vi "Sort_String_Array.vi"(0 "Unsorted String":string[](array[string])) -> (1 "Sorted String":string[](array[string]), 2 "Array 2":dbl[](array[numeric]))   [LabVIEW 2014]
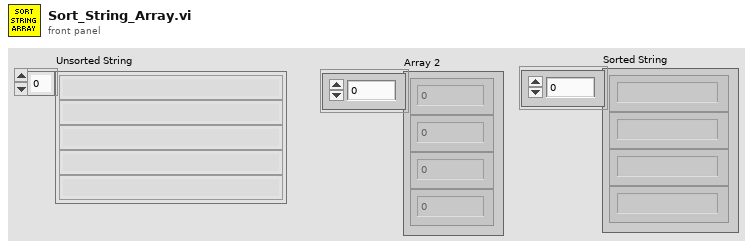
[diagram p1: front panel]
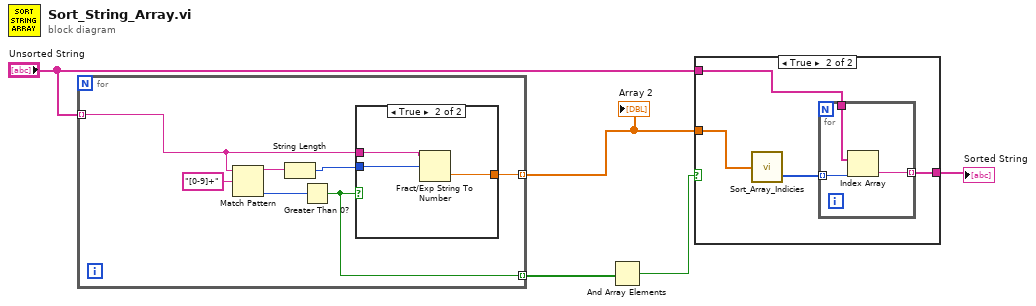
[diagram p0: block diagram]
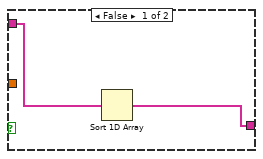
[diagram p2: hidden frame]
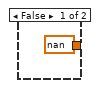
[diagram p3: hidden frame]
diagram:
  n1 = for {
    tunnel: "Unsorted String" -> [w8] mode=indexing
    tunnel: [w7] -> w3 mode=indexing
    tunnel: [w6] -> w2 mode=indexing
    n2 = Match Pattern(string=w8, regular expression="[0-9]+") -> (before substring=w10:string, offset past match=w11:i32)  [unwired: 1 in, 2 out]
    n3 = String Length(string=w10) -> (length=w9:i32)
    n4 = Greater Than 0?(x=w11) -> (x > 0?=w6:bool)
    n5 = case shown="True" w6 {
      tunnel: w9 -> [_ w16]
      tunnel: w8 -> [_ w15]
      tunnel: [nan w14] -> w7
      frame False {
      }
      frame True {
        n6 = Fract/Exp String To Number(string=w15, offset=w16) -> (number=w14:dbl)  [unwired: 3 out]
      }
    }
  }
  "Array 2" <- w3
  n7 = And Array Elements(Boolean array=w2) -> (logical AND=w1:bool)
  n8 = case shown="True" w1 {
    tunnel: w3 -> [_ w22]
    tunnel: "Unsorted String" -> [w18 w20]
    tunnel: [w17 w19] -> w4
    frame False {
      n9 = Sort 1D Array(array=w18) -> (sorted array=w17:string[])
    }
    frame True {
      n10 = call "Sort_Array_Indicies.vi"("unsorted array"=w22) -> ("Sort Index"=w21:i32[])  [unwired: 1 out]
      n11 = for {
        tunnel: w21 -> [w25] mode=indexing
        tunnel: w20 -> [w24]
        tunnel: [w23] -> w19 mode=indexing
        n12 = Index Array(array=w24, index=w25) -> (element=w23:string)
      }
    }
  }
  "Sorted String" <- w4
